vi "IMS  RS232_Comm.vi"(5 "VISA resource name":refnum<visa-resource-name>="COM1", 6 "Delay before Readback(ms)":u32=50, 8 "error in (no error)":errorcluster, 11 "Command String (`\\' Codes Display)":string) -> (0 "error out":errorcluster, 2 "Response (normal display)":string, 3 "data received":bool)   [LabVIEW 2009]
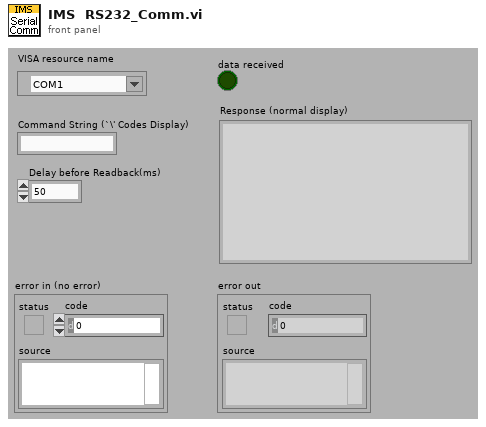
[diagram p1: front panel]
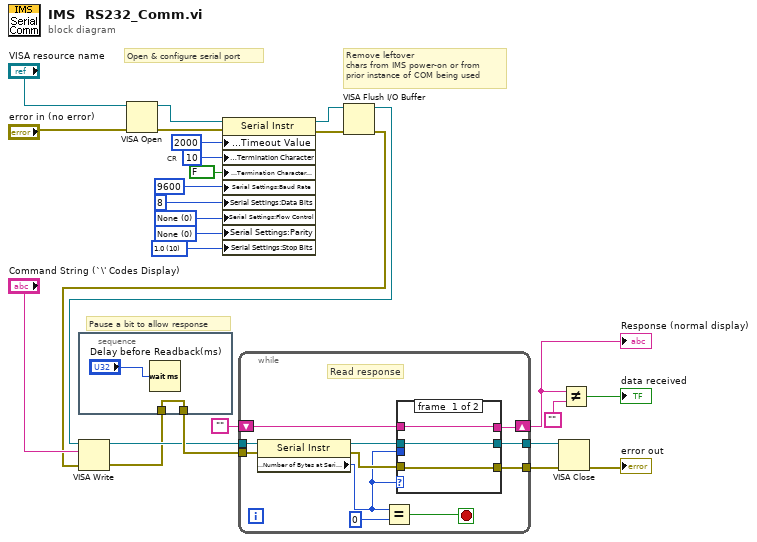
[diagram p0: block diagram]
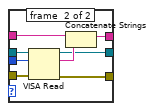
[diagram p2: hidden frame]
diagram:
  w15 = u16 10 items=["1.0"=10, "1.5"=15, "2.0"=20] ("Serial Settings:Serial Stop Bits")
  w14 = u16 0 items=["None", "Odd", "Even", "Mark", "Space"] ("Serial Settings:Serial Parity")
  w13 = u16 0 items=["None", "XON/XOFF", "RTS/CTS", "XON/XOFF & RTS/CTS", "DTR/DSR", "XON/XOFF & DTR/DSR"] ("Serial Settings:Serial Flow Control")
  # "Open & configure serial port"
  # "Remove leftover\nchars from IMS power-on or from\nprior instance of COM being used"
  # "CR"
  # "Pause a bit to allow response"
  n1 = VISA Open(error in (no error)="error in (no error)", VISA resource name="VISA resource name") -> (VISA resource name=w10:refnum<visa-resource-name>, error out=w9:errorcluster)  [unwired: 3 in]
  n2 = property class="Serial Instr"(reference=w10, error in=w9, "General Settings:Timeout Value"=u32 2000, "Message Based Settings:Termination Character"=u8 10, "Message Based Settings:Termination Character Enable"=FALSE, "Serial Settings:Baud Rate"=u32 9600, "Serial Settings:Data Bits"=u16 8 ("Serial Settings:Serial Data Bits"), "Serial Settings:Flow Control"=w13, "Serial Settings:Parity"=w14, "Serial Settings:Stop Bits"=w15) -> (reference out=w16:refnum<visa-resource-name>, error out=w17:errorcluster)
  n3 = VISA Flush I/O Buffer(VISA resource name=w16, error in (no error)=w17) -> (VISA resource name out=w2:refnum<visa-resource-name>, error out=w1:errorcluster)  [unwired: 1 in]
  n4 = VISA Write(VISA resource name=w2, write buffer="Command String (`\\' Codes Display)", error in (no error)=w1) -> (VISA resource name out=w24:refnum<visa-resource-name>, error out=w23:errorcluster)  [unwired: 1 out]
  n5 = stacked-sequence {
    tunnel: w23 -> [w29]
    tunnel: [w29] -> w26
    frame #0 {
      n6 = Wait (ms)(milliseconds to wait="Delay before Readback(ms)") -> ()  [unwired: 1 out]
    }
  }
  n7 = while {
    tunnel: w24 -> [w40]
    tunnel: [w32] -> w4
    tunnel: [w33] -> w5
    tunnel: w26 -> [w39]
    shift-right: [w36] -> w20
    shift-left: "" -> [w35]
    stop <- w37 stop-if-true
    # "Read response"
    n8 = property class="Serial Instr"(reference=w40, error in=w39) -> (reference out=w31:refnum<visa-resource-name>, error out=w34:errorcluster, "Serial Settings:Number of Bytes at Serial Port"=w30:u32)
    n9 = Equal?(x=w30, y=u32 0) -> (x = y?=w37:bool)
    n10 = case shown="1, Default" w30 {
      tunnel: [w43 w51] -> w36
      tunnel: w35 -> [w43 w50]
      tunnel: w34 -> [w41 w49]
      tunnel: [w41 w47] -> w33
      tunnel: [w42 w46] -> w32
      tunnel: w31 -> [w42 w45]
      tunnel: w30 -> [_ w44]
      frame #0 {
      }
      frame #1 {
        n11 = VISA Read(VISA resource name=w45, byte count=w44, error in (no error)=w49) -> (VISA resource name out=w46:refnum<visa-resource-name>, read buffer=w48:string, error out=w47:errorcluster)  [unwired: 1 out]
        n12 = Concatenate Strings(w50, w48) -> (w51:string)
      }
    }
  }
  "Response (normal display)" <- w20
  n13 = VISA Close(VISA resource name=w4, error in (no error)=w5) -> (error out=→"error out":errorcluster)
  n14 = Not Equal?(x=w20, y="") -> (x != y?=→"data received":bool)
